vi "Main App Name.vi"(3 "Apps Name":string="HV60D LV apps Ver 4.0") -> ()   [LabVIEW 2018]
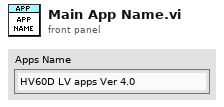
[diagram p1: front panel]
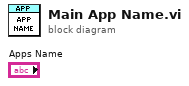
[diagram p0: block diagram]
diagram:
